vi "Create Chans.vi"(5 "New Section Name (none)":string, 6 "new section GUID (\"\":del prot)":string, 7 "Type":T3=enum."Output", 8 "error in (no error)":errorcluster, 10 "Channels":T2[](array[typedef]), 11 "Section Ptr":T1 format="%.0x") -> (0 "error out":errorcluster, 1 "new channel references":T1[](array[typedef]) format="%.0x", 2 "new section ref":T1=18446744073709551615 format="%.0x", 3 "Section Ptr dup":T1 format="%.0x")   [LabVIEW 2015, in "Engine Simulation Toolkit System Explorer.lvlib"]
uses:
  Engine Simulation Toolkit System Explorer.lvlib
  <vilib>/NI Veristand/Custom Device API/Custom Device Item Ref.ctl
  <vilib>/NI Veristand/Custom Device API/Custom Device Channel Type.ctl
  Shared/Channel.ctl
  <vilib>/NI Veristand/Custom Device API/Custom Device Channel.ctl
  Shared/Constants and GUIDs.vi
  <vilib>/NI Veristand/Custom Device API/Custom Device API.lvlib
  Shared/Engine Simulation Toolkit Shared.lvlib
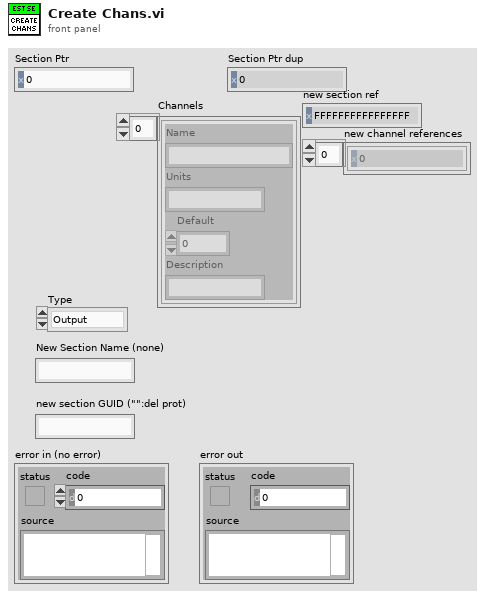
[diagram p1: front panel]
types:
  T1 = typedef "Custom Device API.lvlib/Custom Device Item Ref.ctl" = u64
  T2 = typedef "Engine Simulation Toolkit Shared.lvlib/Channel.ctl" = cluster{"Name":string, "Units":string, "Default":dbl, "Description":string}
  T3 = typedef "Custom Device API.lvlib/Custom Device Channel Type.ctl" = enum16{"Input", "Output"}
  T4 = typedef "Custom Device API.lvlib/Custom Device Channel.ctl" = cluster{"Type":T3, "Units":string, "Default Value":dbl, "Faultable":bool, "Scalable":bool}
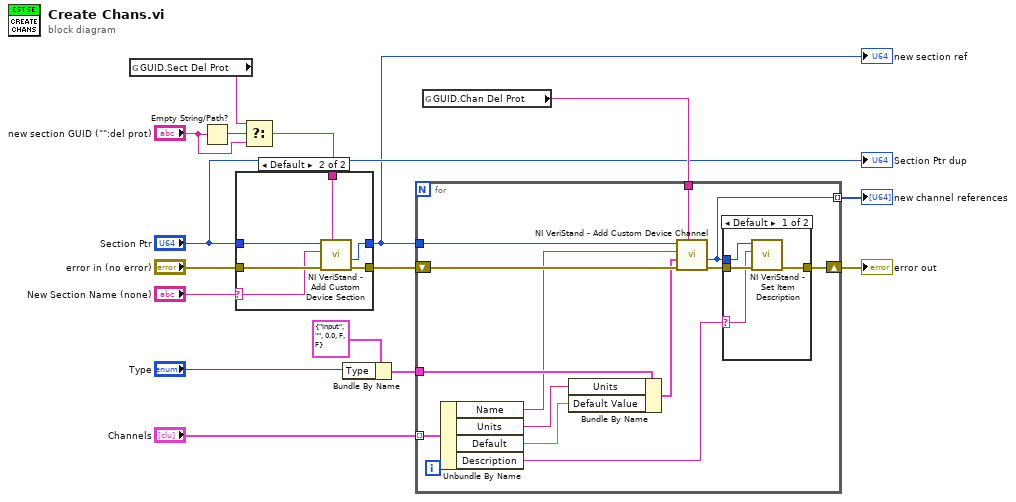
[diagram p0: block diagram]
diagram:
  n1 = global read "Constants and GUIDs.vi" "GUID.Sect Del Prot"() -> (w4:string)
  n2 = Empty String/Path?(string/path="new section GUID (\"\":del prot)") -> (empty?=w5:bool)
  n3 = Select(t=w4, s=w5, f="new section GUID (\"\":del prot)") -> (s? t:f=w2:string)
  n4 = case shown="Default" "New Section Name (none)" {
    selector: "New Section Name (none)" -> [_ w20]
    tunnel: "error in (no error)" -> [w18 w24]
    tunnel: "Section Ptr" -> [w17 w23]
    tunnel: [w18 w22] -> w9
    tunnel: [w17 w21] -> w8
    tunnel: w2 -> [_ w19]
    frame "" {
    }
    frame Default {
      n5 = call <vilib>:"NI VeriStand - Add Custom Device Section.vi"("GUID (Default Section)"=w19, "error in (no error)"=w24, "Section Name"=w20, "Parent Ref in"=w23) -> ("error out"=w22:errorcluster, "Section Ptr"=w21:T1)  [unwired: 4 in, 2 out]
    }
  }
  "new section ref" <- w8
  n6 = Bundle By Name(cluster=T4 {"Type"=enum."Input", "Units"="", "Default Value"=0.0, "Faultable"=FALSE, "Scalable"=FALSE} ("Channel"), "Type"="Type") -> (w10:T4)
  n7 = global read "Constants and GUIDs.vi" "GUID.Chan Del Prot"() -> (w16:string)
  n8 = for {
    tunnel: w8 -> [w36]
    shift-right: [w32] -> w14
    shift-left: w9 -> [w37]
    tunnel: w10 -> [w35]
    tunnel: w16 -> [w33]
    tunnel: "Channels" -> [w30] mode=indexing
    tunnel: [w25] -> w1 mode=indexing
    n9 = Unbundle By Name(w30) -> ("Name"=w29:string, "Units"=w28:string, "Default"=w27:dbl, "Description"=w26:string)
    n10 = Bundle By Name(cluster=w35, "Units"=w28, "Default Value"=w27) -> (w34:T4)
    n11 = call <vilib>:"NI VeriStand - Add Custom Device Channel.vi"("GUID (Default Channel)"=w33, "error in (no error)"=w37, "Channel"=w34, "Channel Name"=w29, "Parent Ref in"=w36) -> ("error out"=w31:errorcluster, "Channel Ref"=w25:T1)  [unwired: 3 in, 2 out]
    n12 = case shown="Default" w26 {
      selector: w26 -> [w38 _]
      tunnel: [w40 w42] -> w32
      tunnel: w31 -> [w41 w42]
      tunnel: w25 -> [w39 _]
      frame Default {
        n13 = call <vilib>:"NI VeriStand - Set Item Description.vi"("error in (no error)"=w41, "Description"=w38, "Item Ref in"=w39) -> ("error out"=w40:errorcluster)  [unwired: 6 in, 2 out]
      }
      frame "" {
      }
    }
  }
  "error out" <- w14
  "new channel references" <- w1
  "Section Ptr dup" <- "Section Ptr"
